vi "SendTo_Notifier.vi"(10 "Message":variant, 11 "Queue Name":string) -> (3 "Node Out":refnum<class "bt_Node.lvclass">)   [LabVIEW 2021, in "BT.lvlib"]
uses:
  BT.lvlib
  Support/Nodes/abs_Node/bt_Node.lvclass
  Support/Nodes/Leaves/Synch/Notifier/Send/bt_Send_Notifier.lvclass
  C:/Users/Tim/Documents/GitHub/LV_Behaviour_Tree/Source/Support/Nodes/Leaves/Synch/With Values/Send/bt_Send_Synch_WithValues.lvclass
  C:/Users/Tim/Documents/GitHub/LV_Behaviour_Tree/Source/Support/Nodes/abs_Node/bt_Node.lvclass
  Support/Nodes/Leaves/Synch/With Values/Send/bt_Send_Synch_WithValues.lvclass/bt_Send_Synch_WithValues.ctl
  Support/Nodes/Leaves/Synch/Notifier/Send/bt_Send_Notifier.lvclass/bt_Send_Notifier.ctl
  Support/Nodes/Leaves/Synch/With Values/Send/Properties/Write Values.vi
  Support/Nodes/Leaves/Synch/Notifier/Send/Properties/Write Name.vi
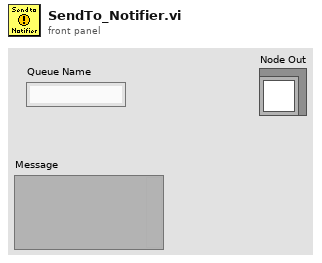
[diagram p1: front panel]
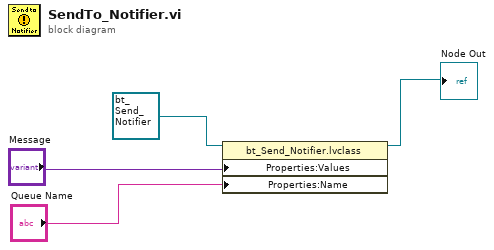
[diagram p0: block diagram]
diagram:
  n1 = property class="bt_Send_Notifier.lvclass"(reference=refnum<class "bt_Send_Notifier.lvclass"> refnum ("BT.lvlib:bt_Send_Notifier.lvclass"), "Properties:Values"="Message", "Properties:Name"="Queue Name") -> (reference out=→"Node Out":refnum<class "bt_Send_Notifier.lvclass">)  [unwired: 1 in, 1 out]
